vi "StandaloneDataAcquisitionTester.vi"() -> ()   [LabVIEW 2018, in "SensorPlugins.lvlib" / "RoomAlert.lvclass"]
uses:
  RoomAlert.lvclass
  Visualization/VisualizeSensor/VisualizeSensor.lvclass
  TypeDefinitions/MeasurementControls.ctl
panel:
  out "MeasurementCluster":T1={"Measurement RefreshTime (ms)"=0, "Measurement Name"="", "Timeout(ms)"=1000, "Amber Warning Light Configuration"={"Warning Temperture (Degrees C)"=0.0, "Temperature Delta (Degrees C/Minute)"=0.0, "Time Window (Minutes)"=0.0}} {"Timeout(ms)" min=1000; "Measurement RefreshTime (ms)" min=1000}
  out "Siemens":waveform(dbl)[](graph)=[{"t0"=timestamp(3657200531.6397257 s since 1904-01-01), "dt"=1.0, "Y"=[46.19]}, {"t0"=timestamp(3657200531.6397257 s since 1904-01-01), "dt"=1.0, "Y"=[2.0]}, {"t0"=timestamp(3657200531.6397257 s since 1904-01-01), "dt"=1.0, "Y"=[60.0]}]
  in  "Boolean":bool
  in  "PluginIniFilePath":path=path "C:/Users/Public/Projects/ICDAS/UserFiles/Plugins/Sensor/RoomAlert/RoomAlert12E-MAC-4125.ini"
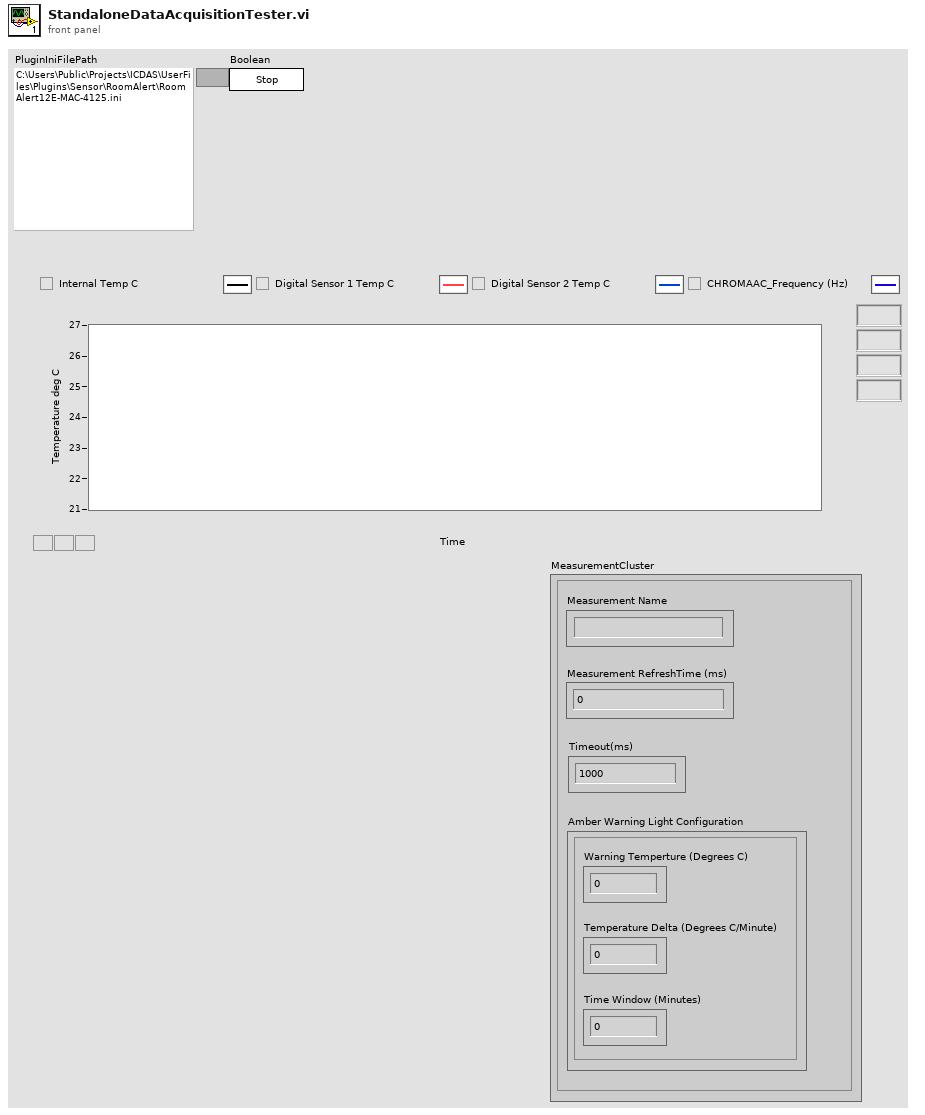
[diagram p1: front panel]
types:
  T1 = typedef "SensorPlugins.lvlib/RoomAlert.lvclass/MeasurementControls.ctl" = cluster{"Measurement RefreshTime (ms)":u32, "Measurement Name":string, "Timeout(ms)":i32, "Amber Warning Light Configuration":cluster{"Warning Temperture (Degrees C)":dbl, "Temperature Delta (Degrees C/Minute)":dbl, "Time Window (Minutes)":dbl}}
  T2 = typedef "SensorShared.lvlib/clSensorData.ctl" = cluster{"SensorType":string, "SensorData":variant}
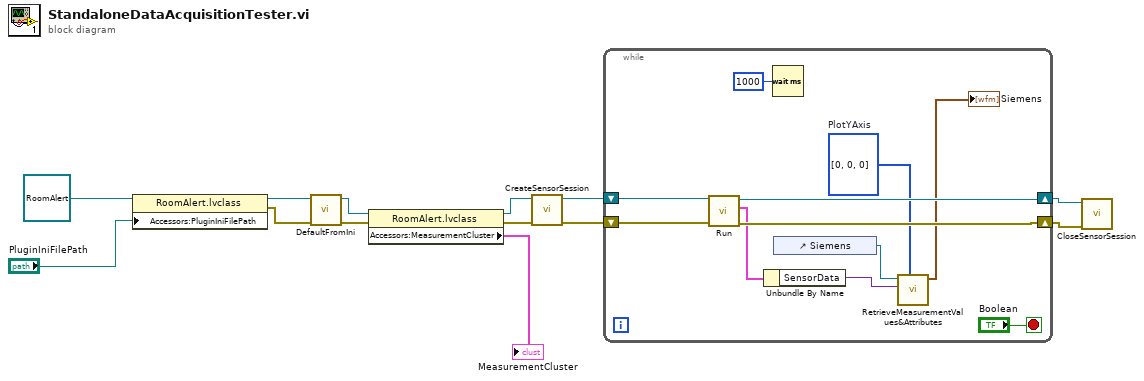
[diagram p0: block diagram]
diagram:
  n1 = property class="RoomAlert.lvclass"(reference=refnum<class "RoomAlert.lvclass"> refnum ("SensorPlugins.lvlib:RoomAlert.lvclass"), "Accessors:PluginIniFilePath"="PluginIniFilePath") -> (reference out=w12:refnum<class "RoomAlert.lvclass">, error out=w9:errorcluster)  [unwired: 1 in]
  n2 = call-dynamic "DefaultFromIni.vi"("error in (no error)"=w9, "RoomAlert in"=w12) -> ("error out"=w10:errorcluster, "RoomAlert out"=w3:refnum<class "RoomAlert.lvclass">)  [unwired: 8 in]
  n3 = property class="RoomAlert.lvclass"(reference=w3, error in=w10) -> (reference out=w2:refnum<class "RoomAlert.lvclass">, error out=w4:errorcluster, "Accessors:MeasurementCluster"=→"MeasurementCluster":T1)
  n4 = call-dynamic "CreateSensorSession.vi"("error in (no error)"=w4, "RoomAlert in"=w2) -> ("error out"=w7:errorcluster, "RoomAlert out"=w8:refnum<class "RoomAlert.lvclass">)  [unwired: 8 in]
  n5 = while {
    shift-right: [w20] -> w6
    shift-left: w8 -> [w22]
    shift-right: [w19] -> w5
    shift-left: w7 -> [w21]
    stop <- "Boolean" stop-if-true
    w16 = u32[] [0, 0, 0]  # PlotYAxis
    n6 = call-dynamic "Run.vi"("error in (no error)"=w21, "RoomAlert in"=w22) -> ("error out"=w19:errorcluster, "clSensorData"=w15:T2, "RoomAlert out"=w20:refnum<class "RoomAlert.lvclass">)  [unwired: 6 in, 1 out]
    n7 = Unbundle By Name(w15) -> ("SensorData"=w17:variant)
    n8 = Wait (ms)(milliseconds to wait=u32 1000) -> ()  [unwired: 1 out]
    n9 = control-ref of="Siemens"() -> (w18:refnum<vi>)
    n10 = call "RetrieveMeasurementValues&Attributes.vi"("PlotYScale"=w16, "Variant"=w17, "WaveformChartReference"=w18) -> ("WaveformArrayOut"=→"Siemens":waveform(dbl)[])  [unwired: 4 in, 4 out]
  }
  n11 = call-dynamic "CloseSensorSession.vi"("error in (no error)"=w5, "RoomAlert in"=w6) -> ()  [unwired: 8 in, 2 out]
